vi "Do.vi"(8 "error in":errorcluster, 10 "Actor in":refnum<class "Actor.lvclass">, 11 "Update PMT Gains MSG":refnum<class "Update PMT Gains MSG.lvclass">) -> (0 "error out":errorcluster, 2 "Actor out":refnum<class "Actor.lvclass">)   [LabVIEW 2014, in "eCRDS Library.lvlib" / "Update PMT Gains MSG.lvclass"]
doc: "(<B>Filename</B>: Actor Framework.lvlib:Message.lvclass:Do.vi)\n\nDefines what a message does when it is received by an actor. Generally, a message instructs an actor to invoke one of its methods. By default, this method does nothing. A child class must override it to define behavior. Create a child class by using the Actor Framework Message Maker dialog box."
uses:
  Update PMT Gains MSG.lvclass
  <vilib>/ActorFramework/Actor/Actor.lvclass
  Update PMT Gains MSG.lvclass/Update PMT Gains MSG.ctl
  Instr Actor.lvclass
  Instr Actor.lvclass/Instr Actor.ctl
  Controller/Messages/Update CVT/Update CVT Data.lvclass
  Controller/Messages/Update CVT/Update CVT Data.lvclass/Update CVT Data.ctl
  Controller/Messages/Update CVT/Write Data.vi
  Controller/Messages/Update CVT/Write Group.vi
  Controller/Messages/Update CVT/Write tag.vi
  <vilib>/DAQmx/write.llb/DAQmx Write (Analog 1D DBL NChan 1Samp).vi
  reusable/Session APIs/Session Log/System Log.lvclass
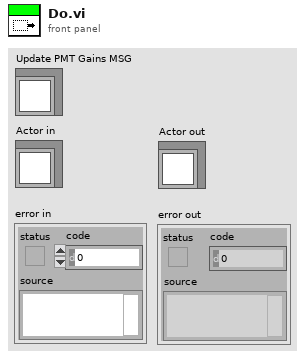
[diagram p1: front panel]
types:
  T1 = typedef "Session - Root.lvclass/Session Handle.ctl" = refnum<data-value>
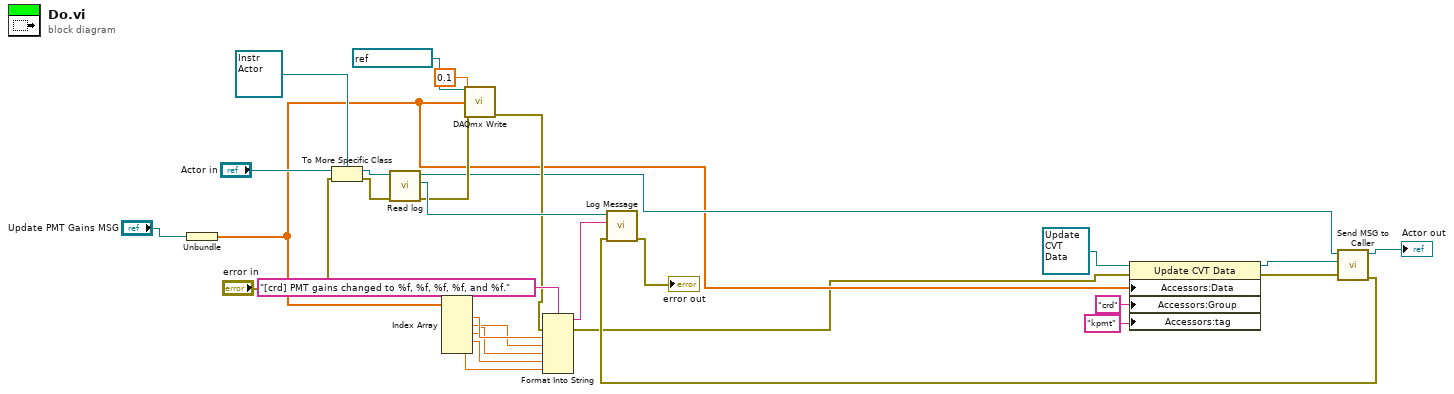
[diagram p0: block diagram]
diagram:
  n1 = Unbundle("Update PMT Gains MSG") -> (w3:dbl[])
  n2 = To More Specific Class(target class=refnum<class "Instr Actor.lvclass"> refnum ("Instrument Lib:Instr"), reference="Actor in", error in="error in") -> (specific class reference=w25:refnum<class "Instr Actor.lvclass">, error out=w20:errorcluster)
  n3 = call "Read log.vi"("error in (no error)"=w20, "Instr Actor in"=w25) -> ("error out"=w19:errorcluster, "Session Handle"=w24:T1, "Instr Actor out"=w5:refnum<class "Instr Actor.lvclass">)  [unwired: 7 in]
  n4 = Index Array(array=w3) -> (element #1=w18:dbl, element #2=w16:dbl, element #3=w15:dbl, element #4=w14:dbl, element #5=w13:dbl)  [unwired: 5 in]
  n5 = call-poly <vilib>:"DAQmx Write.vi"("task/channels in"=refnum<k21> "PMT Gain", "data"=w3, "timeout"=0.1, "error in"=w19) -> ("error out"=w11:errorcluster)  [unwired: 9 in, 2 out]
  n6 = Format Into String(format string="[crd] PMT gains changed to %f, %f, %f, %f, and %f.", error in=w11, w18, w16, w15, w14, w13) -> (resulting string=w12:string, error out=w1:errorcluster)  [unwired: 1 in]
  n7 = property class="Update CVT Data"(reference=refnum<class "Update CVT Data.lvclass"> refnum ("Controller.lvlib:Update CVT Data"), error in=w1, "Accessors:Data"=w3, "Accessors:Group"="crd" ("Group"), "Accessors:tag"="kpmt" ("tag")) -> (reference out=w7:refnum<class "Update CVT Data.lvclass">, error out=w6:errorcluster)
  n8 = call "Send MSG to Caller.vi"("error in"=w6, "Message"=w7, "Instr in"=w5) -> ("error out"=w2:errorcluster, "Instr out"=→"Actor out":refnum<class "Instr Actor.lvclass">)  [unwired: 7 in]
  n9 = call "Log Message.vi"("error in"=w2, "MSG In"=w12, "session in"=w24) -> ("error out"=→"error out":errorcluster)  [unwired: 7 in, 1 out]
